vi "XYGraphLogGen.vi"(0 "NouvTemps":dbl, 1 "XData":dbl[](array[numeric]) caption="Tout les DonnX", 2 "TracerCourbe":bool[](array[boolean]), 5 "AllXYGraphIn":T1(array[cluster]), 7 "NouvDonnées Y":dbl[](array[numeric]), 9 "Actual Point Index":i32, 11 "error in (no error)":errorcluster, 12 "All YData":dbl[][](array[numeric]), 13 "Max Index":i32) -> (3 "XData Out":dbl[](array[numeric]) caption="Tout les DonnX Out", 6 "AllXYGraphOut":T1(array[cluster]), 8 "XYGraph":T1(array[cluster]), 14 "All YData out":dbl[][](array[numeric]), 15 "error out":errorcluster)   [LabVIEW 2010]
doc: "Ce Vi ajoute les nouvelles données acquisitionner dans les tables de toutes les données acquisitionner. Il formate ensuite les données sous forme de cluster pour l'affichage dans un graphique XY."
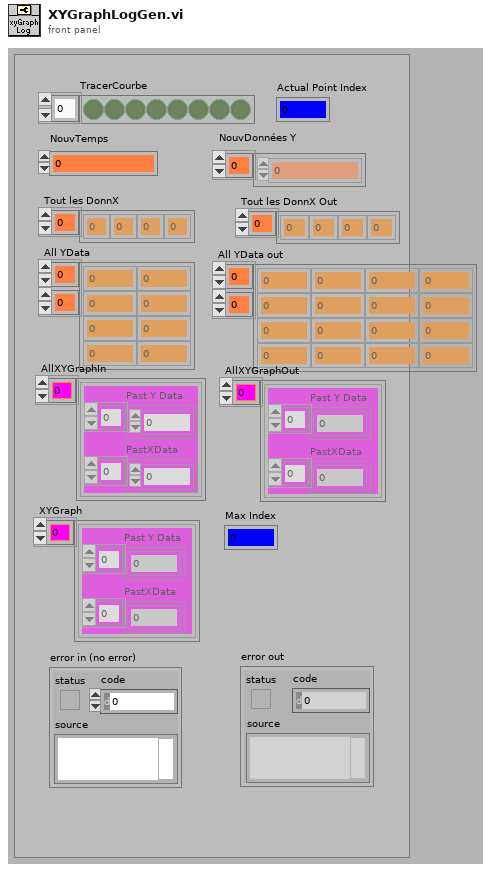
[diagram p1: front panel]
types:
  T1 = cluster{"Past Y Data":dbl[], "PastXData":dbl[]}[]
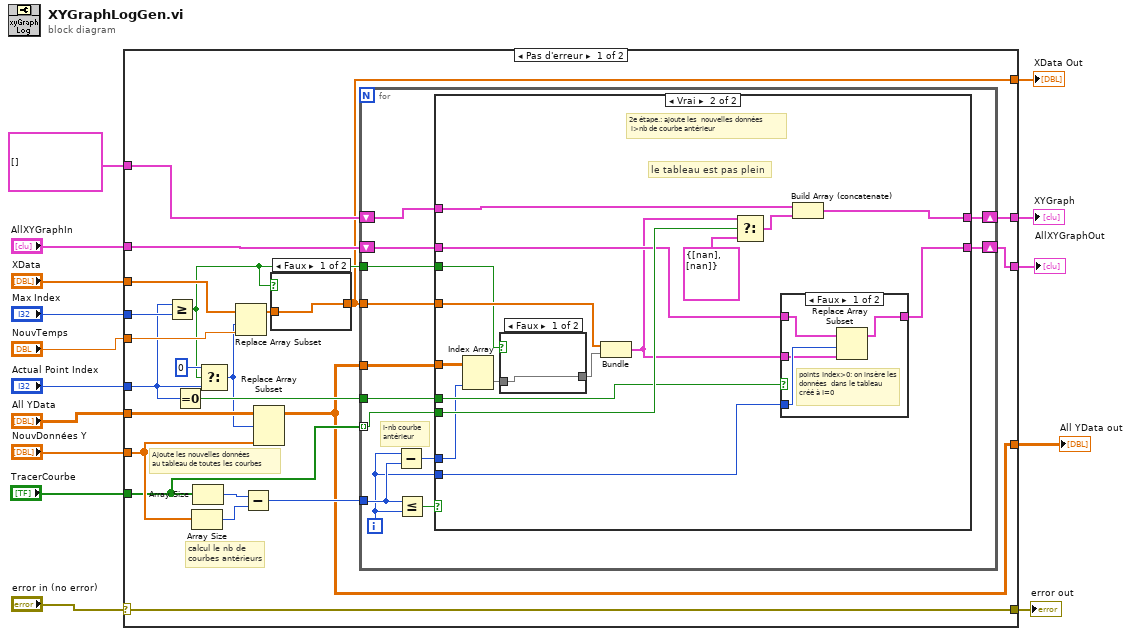
[diagram p0: block diagram]
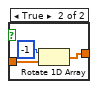
[diagram p2: hidden frame]
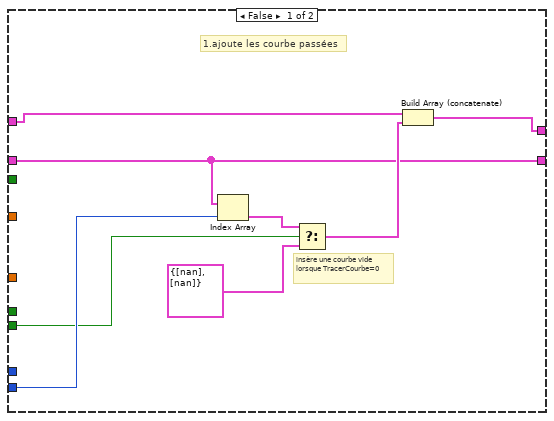
[diagram p3: hidden frame]
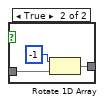
[diagram p4: hidden frame]
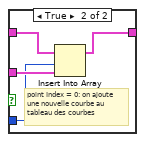
[diagram p5: hidden frame]
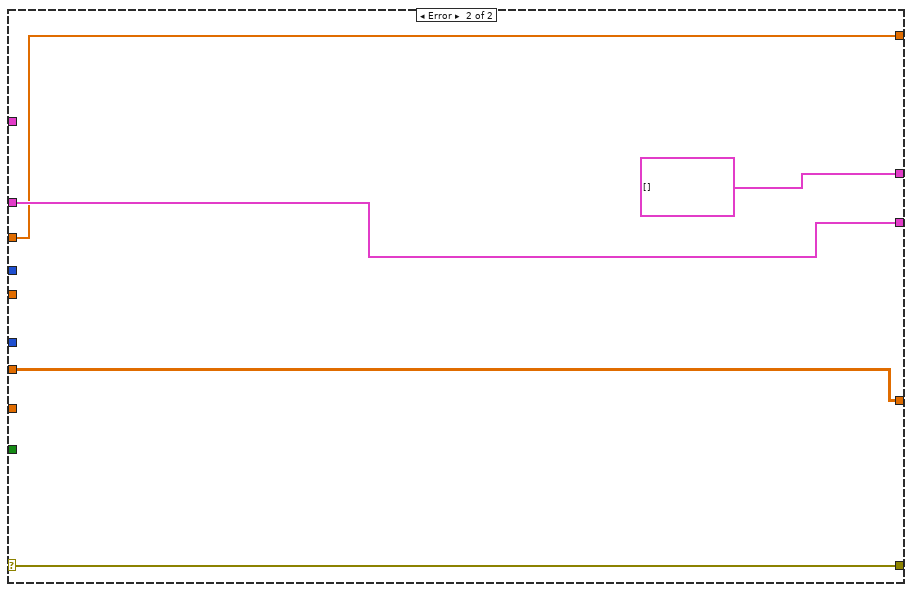
[diagram p6: hidden frame]
diagram:
  n1 = case shown="Pas d'erreur" "error in (no error)" {
    selector: "error in (no error)" -> [w36 w95]
    tunnel: "NouvDonnées Y" -> [w28 _]
    tunnel: "XData" -> [w22 w91]
    tunnel: "NouvTemps" -> [w32 _]
    tunnel: "Actual Point Index" -> [w18 _]
    tunnel: "All YData" -> [w33 w92]
    tunnel: [w34 cluster{"XData":dbl[], "All YData":dbl[]}[] []] -> w10
    tunnel: [w36 w95] -> w11
    tunnel: [w19 w91] -> w1
    tunnel: T1 [] ("XYGraph In") -> [w37 _]
    tunnel: "Max Index" -> [w35 _]
    tunnel: "TracerCourbe" -> [w24 _]
    tunnel: "AllXYGraphIn" -> [w27 w93]
    tunnel: [w26 w93] -> w3
    tunnel: [w16 w92] -> w2
    frame No Error {
      # "calcul le nb de courbes antérieurs"
      # "Ajoute les nouvelles données\nau tableau de toutes les courbes"
      n2 = Greater Or Equal?(x=w18, y=w35) -> (x >= y?=w21:bool)
      n3 = Equal To 0?(x=w18) -> (x = 0?=w23:bool)
      n4 = Array Size(array=w28) -> (size(s)=w30:i32)
      n5 = Array Size(array=w24) -> (size(s)=w31:i32)
      n6 = Select(t=0 ("disabled index (col)"), s=w21, f=w18) -> (s? t:f=w17:i32)
      n7 = Replace Array Subset(array=w22, new element=w32, index=w17) -> (w20:dbl[])
      n8 = Subtract(x=w31, y=w30) -> (x-y=w29:i32)
      n9 = Replace Array Subset(array=w33, new element=w28, index (row)=w17) -> (w16:dbl[][])  [unwired: 1 in]
      n10 = case shown="Faux" w21 {
        tunnel: w20 -> [w38 w39]
        tunnel: [w38 w40] -> w19
        frame False {
        }
        frame True {
          n11 = Rotate 1D Array(1:w39, 2:-1 ("n")) -> (0:w40:dbl[])
        }
      }
      n12 = for {
        tunnel: w24 -> [w45] mode=indexing
        tunnel: w19 -> [w53]
        tunnel: w21 -> [w52]
        shift-right: [w51] -> w34
        shift-left: w37 -> [w54]
        tunnel: w16 -> [w50]
        tunnel: w29 -> [w49]
        shift-right: [w46] -> w26
        shift-left: w27 -> [w47]
        tunnel: w23 -> [w43]
        i -> [w48]
        # "i-nb courbe\nantérieur"
        n13 = Subtract(x=w48, y=w49) -> (x-y=w42:i32)
        n14 = Less Or Equal?(x=w49, y=w48) -> (x <= y?=w44:bool)
        n15 = case shown="Vrai" w44 {
          tunnel: w45 -> [w55 w78]
          tunnel: w54 -> [w58 w77]
          tunnel: w53 -> [_ w76]
          tunnel: w52 -> [_ w64]
          tunnel: [w57 w75] -> w51
          tunnel: w50 -> [_ w74]
          tunnel: w48 -> [w60 w73]
          tunnel: w47 -> [w56 w72]
          tunnel: [w56 w70] -> w46
          tunnel: w43 -> [_ w71]
          tunnel: w42 -> [_ w63]
          frame False {
            # "insère une courbe vide lorsque TracerCourbe=0"
            # "1.ajoute les courbe passées"
            n16 = Index Array(array=w56, index=w60) -> (element=w62:cluster{"Past Y Data":dbl[], "PastXData":dbl[]})
            n17 = Select(t=w62, s=w55, f=cluster{"Past Y Data":dbl[], "PastXData":dbl[]} {"Past Y Data"=[nan], "PastXData"=[nan]}) -> (s? t:f=w59:cluster{"Past Y Data":dbl[], "PastXData":dbl[]})
            n18 = Build Array (concatenate)(w58, w59) -> (w57:T1)
          }
          frame True {
            # "le tableau est pas plein"
            # "2e étape.: ajoute les  nouvelles données\n i>nb de courbe antérieur"
            n19 = Index Array(array=w74, index (col)=w63) -> (element=w65:dbl[])  [unwired: 1 in]
            n20 = case shown="Faux" w64 {
              tunnel: [w79 w82] -> w69
              tunnel: w65 -> [w79 w80]
              frame False {
              }
              frame True {
                n21 = Rotate 1D Array(1:w80, 2:-1 ("n")) -> (0:w82:dbl[])
              }
            }
            n22 = Bundle("XData"=w76, "All YData"=w69) -> (w66:cluster{"XData":dbl[], "All YData":dbl[]})  [unwired: 1 in]
            n23 = Select(t=w66, s=w78, f=cluster{"Past Y Data":dbl[], "PastXData":dbl[]} {"Past Y Data"=[nan], "PastXData"=[nan]}) -> (s? t:f=w68:cluster{"Past Y Data":dbl[], "PastXData":dbl[]})
            n24 = case shown="Faux" w71 {
              tunnel: w72 -> [w84 w90]
              tunnel: w66 -> [w85 w89]
              tunnel: [w83 w88] -> w70
              tunnel: w73 -> [w86 w87]
              frame False {
                # "points Index>0: on insère les données  dans le tableau créé à I=0"
                n25 = Replace Array Subset(array=w84, new element=w85, index=w86) -> (w83:T1)
              }
              frame True {
                # "point Index = 0: on ajoute une nouvelle courbe au tableau des courbes"
                n26 = Insert Into Array(array=w90, index=w87, new element=w89) -> (w88:T1)
              }
            }
            n27 = Build Array (concatenate)(w77, w68) -> (w75:T1)
          }
        }
      }
    }
    frame Error {
    }
  }
  "error out" <- w11
  "XYGraph" <- w10
  "All YData out" <- w2
  "XData Out" <- w1
  "AllXYGraphOut" <- w3
